vi "Get Cache User Parameters File Path.vi"(8 "error in (no error)":errorcluster, 11 "Springboard Station Configuration in":refnum<class "Springboard Station Configuration.lvclass">) -> (0 "error out":errorcluster, 2 "station config INI path":path, 3 "Springboard Station Configuration out":refnum<class "Springboard Station Configuration.lvclass">)   [LabVIEW 2022 SP3, in "Springboard TLB`.lvlib" / "Springboard Station Configuration.lvclass"]
uses:
  Springboard Station Configuration.lvclass
  Springboard Station Configuration.lvclass/Springboard Station Configuration.ctl
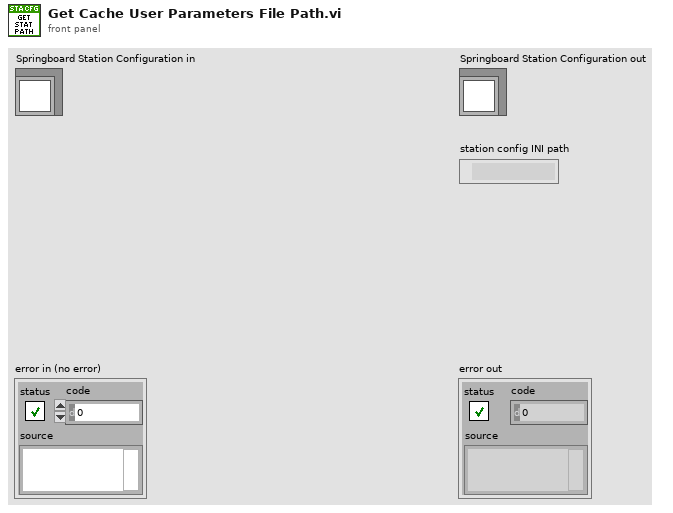
[diagram p1: front panel]
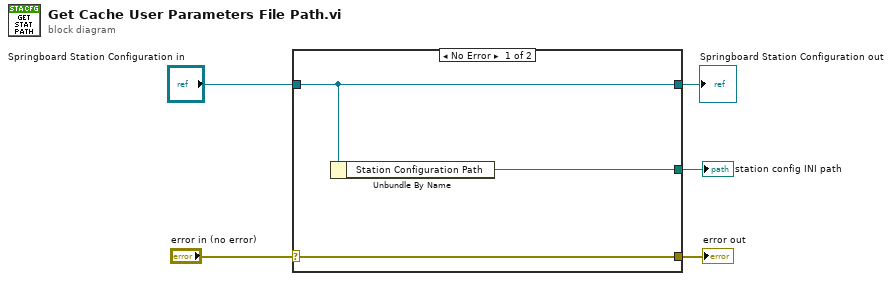
[diagram p0: block diagram]
diagram:
  n1 = case shown="No Error" "error in (no error)" {
    selector: "error in (no error)" -> [w8 w9]
    tunnel: [w8 w9] -> w4
    tunnel: [w7 w10] -> w2
    tunnel: "Springboard Station Configuration in" -> [w7 w10]
    tunnel: [w6 _] -> w1
    frame No Error {
      n2 = Unbundle By Name(w7) -> ("Station Configuration Path"=w6:path)
    }
    frame Error {
    }
  }
  "error out" <- w4
  "Springboard Station Configuration out" <- w2
  "station config INI path" <- w1
